vi "GetParam.vi"(8 "error in (no error)":errorcluster caption="entrée d'erreur (pas d'erreur)", 11 "PowerTransformer.lvclass":refnum<class "PowerTransformer.lvclass">) -> (0 "error out":errorcluster caption="sortie d'erreur", 2 "PowerTransformer":T1={"method"="yeo-johnson", "standardize"=TRUE, "copy"=TRUE}, 3 "PowerTransformer.lvclass":refnum<class "PowerTransformer.lvclass">)   [LabVIEW 2020, in "PowerTransformer.lvclass"]
doc: "Get Parameters"
uses:
  PowerTransformer.lvclass
  PowerTransformer.lvclass/PowerTransformer.ctl
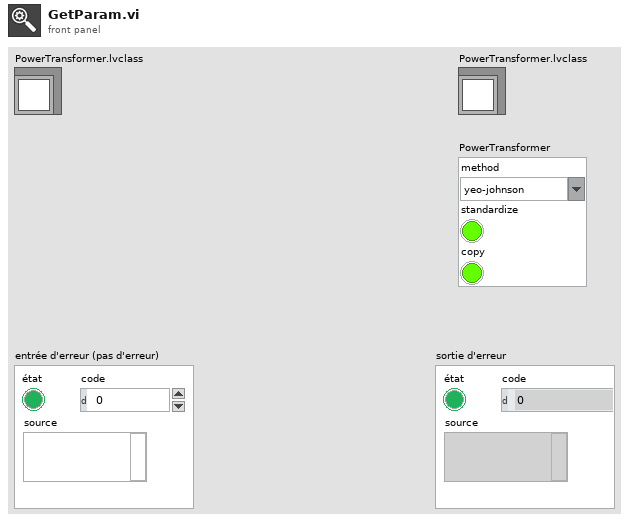
[diagram p1: front panel]
types:
  T1 = cluster{"method":string, "standardize":bool, "copy":bool}
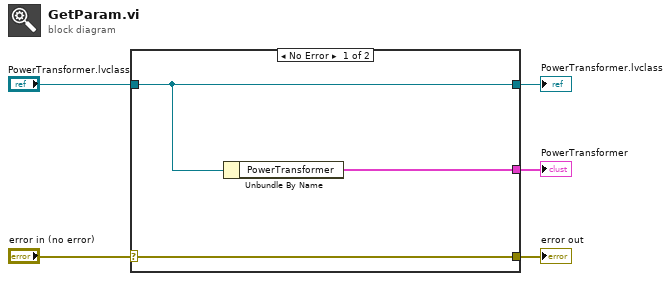
[diagram p0: block diagram]
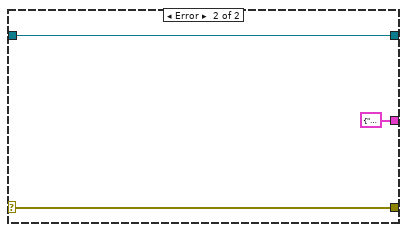
[diagram p2: hidden frame]
diagram:
  n1 = case shown="No Error" "error in (no error)" {
    selector: "error in (no error)" -> [w8 w10]
    tunnel: [w8 w10] -> w4
    tunnel: [w7 w11] -> w2
    tunnel: "PowerTransformer.lvclass" -> [w7 w11]
    tunnel: [w6 T1 {"method"="", "standardize"=FALSE, "copy"=FALSE} ("PowerTransformer")] -> w1
    frame No Error {
      n2 = Unbundle By Name(w7) -> ("PowerTransformer"=w6:T1)
    }
    frame Error {
    }
  }
  "error out" <- w4
  "PowerTransformer.lvclass" <- w2
  "PowerTransformer" <- w1
